vi "Barcode_Reader_Dialog_SoftFP.vi"(0 "reference in":refnum<class "Barcode_Reader_Dialog.lvclass">, 2 "Floating":bool, 5 "error in (no error)":errorcluster) -> (14 "reference out":refnum<class "Barcode_Reader_Dialog.lvclass">, 19 "error out":errorcluster)   [LabVIEW 2022 SP3, in "Barcode_Reader_Dialog.lvlib" / "Barcode_Reader_Dialog.lvclass"]
uses:
  Barcode_Reader_Dialog.lvclass
  Components/ViPER.lvlibp/ViPER.lvclass
  C:/Projects/Medulla/ViPER/Examples/Flux_Capacitor_Tester/Components/ViPER.lvlibp/ViPER.lvclass
panel:
  out "SN":string caption="String"
  in  "Read":bool caption="Blank"
  # "Put your FP UI here"
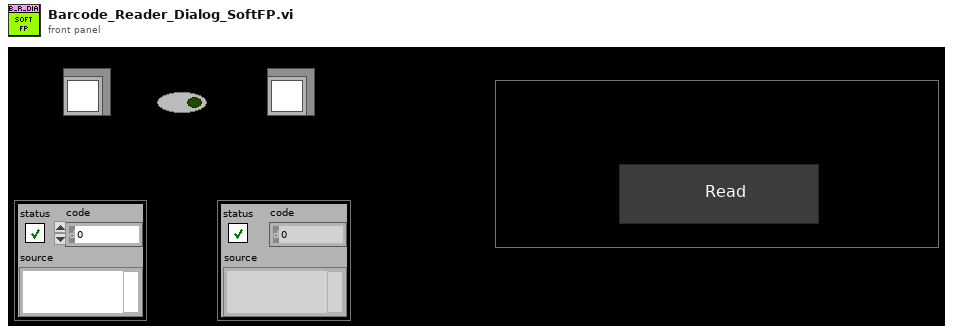
[diagram p1: front panel]
types:
  T1 = enum32{"Invalid", "Standard", "Closed", "Hidden", "Minimized", "Maximized"}
  T2 = typedef "Barcode_Reader_Dialog.lvlib/Barcode_Reader_Dialog.lvclass/ObjectAttributes.ctl" = cluster{"Config":T3, "Serial":string}
  T3 = typedef "Barcode_Reader_Dialog.lvlib/Barcode_Reader_Dialog.lvclass/Config.ctl" = cluster{"default":string}
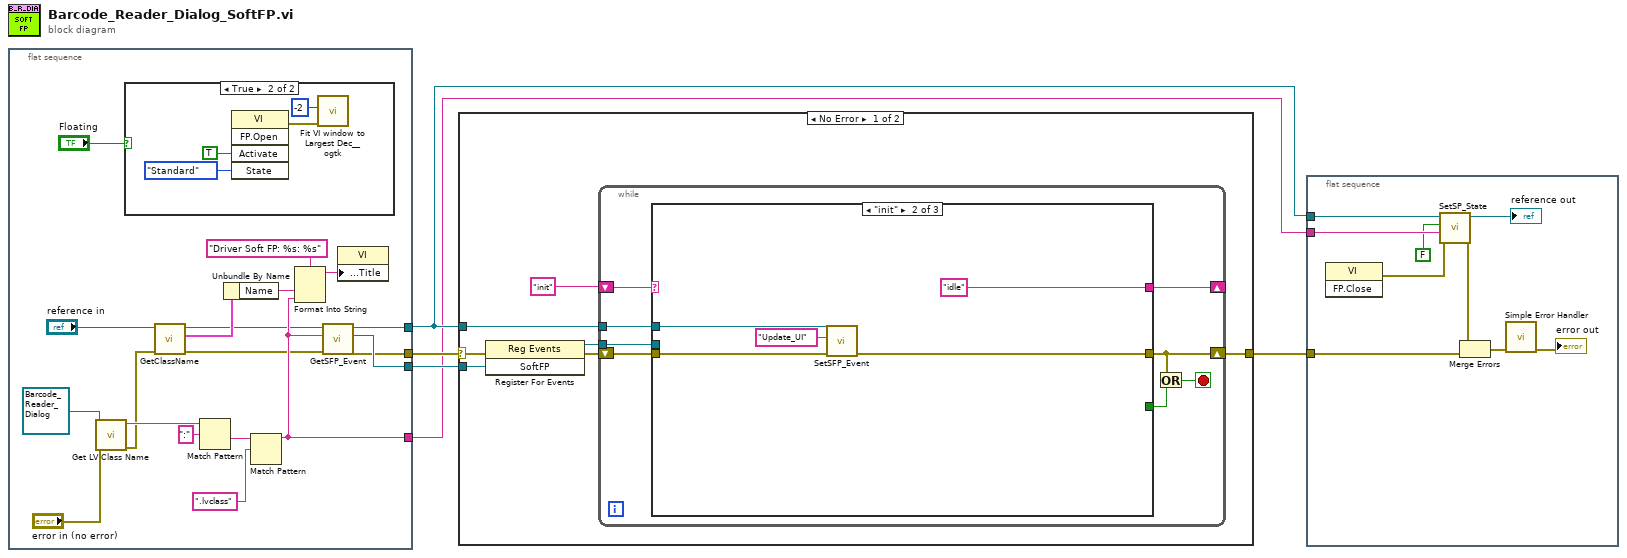
[diagram p0: block diagram]
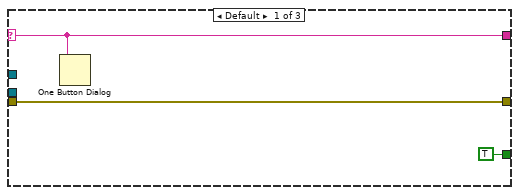
[diagram p3: hidden frame]
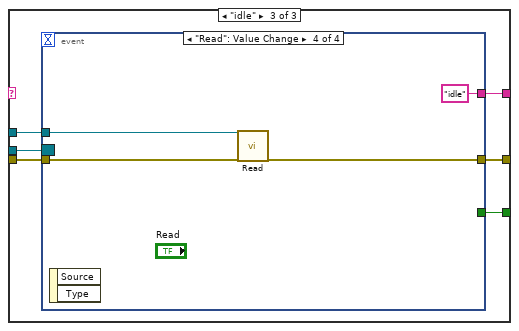
[diagram p4: hidden frame]
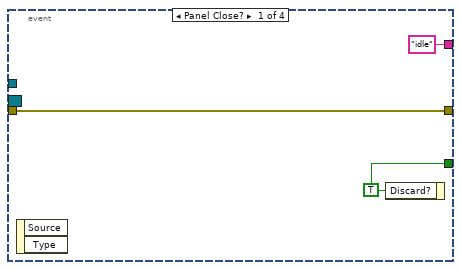
[diagram p5: hidden frame]
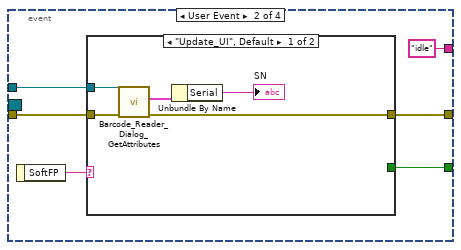
[diagram p6: hidden frame]
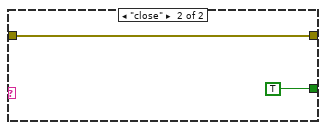
[diagram p7: hidden frame]
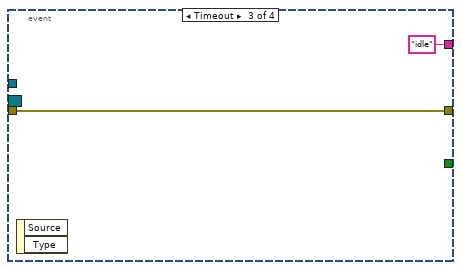
[diagram p8: hidden frame]
diagram:
  n1 = flat-sequence {
    tunnel: [w21] -> w5
    tunnel: [w20] -> w2
    tunnel: [w24] -> w3
    tunnel: [w12] -> w1
    frame #0 {
      n2 = call <vilib>:"Get LV Class Name.vi"("error in (no error)"="error in (no error)", "object"=refnum<class "Barcode_Reader_Dialog.lvclass"> refnum ("reference")) -> ("error out"=w11:errorcluster, "class name"=w17:string)  [unwired: 8 in]
      n3 = case shown="True" "Floating" {
        frame False {
        }
        frame True {
          n4 = invoke class="VI" method="FP.Open"("Activate"=TRUE ("Activate?"), "State"=T1."Standard") -> (error out=w25:errorcluster)  [unwired: 3 in, 4 out]
          n5 = call <userlib>:"Fit VI window to Largest Dec__ogtk.vi"("error in (no error)"=w25, "border spacing (2 px)"=-2) -> ()  [unwired: 4 in, 2 out]
        }
      }
      n6 = call "GetClassName.vi"("error in (no error)"=w11, "reference in"="reference in") -> ("error out"=w10:errorcluster, "Details"=w9:cluster{"Name":string, "Class":string}, "reference out"=w7:refnum<class "Barcode_Reader_Dialog.lvclass">)  [unwired: 7 in]
      n7 = Match Pattern(string=w17, regular expression=":") -> (after substring=w15:string)  [unwired: 1 in, 3 out]
      n8 = Unbundle By Name(w9) -> ("Name"=w19:string)
      n9 = Match Pattern(string=w15, regular expression=".lvclass") -> (before substring=w12:string)  [unwired: 1 in, 3 out]
      n10 = Format Into String(format string="Driver Soft FP: %s: %s", w19, w12) -> (resulting string=w23:string)  [unwired: 2 in, 1 out]
      n11 = call-dynamic "GetSFP_Event.vi"("error in (no error)"=w10, "Ancestor"=w12, "reference in"=w7) -> ("error out"=w21:errorcluster, "SoftFP"=w24:refnum<user-event>, "reference out"=w20:refnum<class "Barcode_Reader_Dialog.lvclass">)  [unwired: 6 in]
      n12 = property class="VI"("Front Panel.Title"=w23) -> ()  [unwired: 2 in, 2 out]
    }
  }
  n13 = case shown="No Error" w5 {
    selector: w5 -> [w33 w80]
    tunnel: [w29 w80] -> w4
    tunnel: w2 -> [w30 _]
    tunnel: w3 -> [w35 _]
    frame No Error {
      n14 = register-events(error in=w33, w35) -> (reference out=w34:refnum<event-registration>, error out=w32:errorcluster)  [unwired: 1 in]
      n15 = while {
        shift-right: [w40] -> w29
        shift-left: w32 -> [w43]
        tunnel: w34 -> [w42]
        tunnel: w30 -> [w41]
        shift-right: [w36] -> _
        shift-left: "init" -> [w37]
        stop <- w39 stop-if-true
        n16 = case shown="\"init\"" w37 {
          selector: w37 -> [w44 _ _]
          tunnel: w43 -> [w45 w48 w57]
          tunnel: w42 -> [_ _ w56]
          tunnel: w41 -> [_ w47 w55]
          tunnel: [w45 w49 w54] -> w40
          tunnel: [TRUE ("Discard?") _ w53] -> w38
          tunnel: [w44 "idle" w52] -> w36
          frame Default {
            n17 = One Button Dialog(message=w44) -> ()  [unwired: 1 in, 1 out]
          }
          frame "init" {
            n18 = call-dynamic "SetSFP_Event.vi"("error in (no error)"=w48, "msg"="Update_UI", "reference in"=w47) -> ("error out"=w49:errorcluster)  [unwired: 7 in, 1 out]
          }
          frame "idle" {
            n19 = event shown="[3] \"Read\": Value Change" {
              selector: w56 -> [_ _ _ _]
              dyn-events: _ -> [_ _ _ _]
              timeout: _ -> [_ _ _ _]
              tunnel: w57 -> [w60 w66 w75 w79]
              tunnel: [w60 w64 w75 w78] -> w54
              tunnel: [w59 w63 _ _] -> w53
              tunnel: w55 -> [_ w61 _ w77]
              tunnel: ["idle" "idle" "idle" "idle"] -> w52
              event Panel Close? {
                w59 = TRUE ("Discard?")
                n20 = event-data() -> ()  [unwired: 1 in, 2 out]
                n21 = event-data("Discard?"=w59) -> ()  [unwired: 1 in, 1 out]
              }
              event User Event {
                n22 = event-data() -> ("SoftFP"=w65:string)  [unwired: 1 in]
                n23 = case shown="\"Update_UI\", Default" w65 {
                  tunnel: w66 -> [w70 w73]
                  tunnel: [w71 w73] -> w64
                  tunnel: [_ TRUE ("Discard?")] -> w63
                  tunnel: w61 -> [w69 _]
                  frame "Update_UI", Default {
                    n24 = call "Barcode_Reader_Dialog_GetAttributes.vi"("error in (no error)"=w70, "reference in"=w69) -> ("error out"=w71:errorcluster, "Data"=w68:T2)  [unwired: 6 in, 2 out]
                    n25 = Unbundle By Name(w68) -> ("Serial"=→"SN":string)
                  }
                  frame "close" {
                  }
                }
              }
              event Timeout {
                n26 = event-data() -> ()  [unwired: 1 in, 2 out]
              }
              event "Read": Value Change {
                n27 = event-data() -> ()  [unwired: 1 in, 2 out]
                n28 = call-dynamic "Read.vi"("reference in"=w77, "error in (no error)"=w79) -> ("error out"=w78:errorcluster)  [unwired: 14 in, 3 out]
              }
            }
          }
        }
        n29 = Or(x=w40, y=w38) -> (x .or. y?=w39:bool)
      }
    }
    frame Error {
    }
  }
  n30 = flat-sequence {
    tunnel: w4 -> [w87]
    tunnel: w2 -> [w82]
    tunnel: w1 -> [w84]
    frame #0 {
      n31 = invoke class="VI" method="FP.Close"() -> (error out=w86:errorcluster)  [unwired: 3 in, 2 out]
      n32 = call "SetSP_State.vi"("error in (no error)"=w86, "Ancestor"=w84, "SP Open"=FALSE, "reference in"=w82) -> ("error out"=w85:errorcluster, "reference out"=→"reference out":refnum<class "Barcode_Reader_Dialog.lvclass">)  [unwired: 6 in]
      n33 = Merge Errors(w85, w87) -> (w89:errorcluster)
      n34 = call <vilib>:"Simple Error Handler.vi"("error in (no error)"=w89) -> ("error out"=→"error out":errorcluster)  [unwired: 4 in, 4 out]
    }
  }
